vi "dfd_Expand Roots.vi"(1 "roots":T1[](array[typedef])) -> (0 "expanded roots":cdb[](array[numeric]))   [LabVIEW 2017, in "NI_DigFilterLicensed.lvlib"]
uses:
  <vilib>/addons/Digital Filter Design/NI_DigFilterLicensed.lvlib
  <vilib>/addons/Digital Filter Design/_Objects.llb/DFD Pole-Zero.ctl
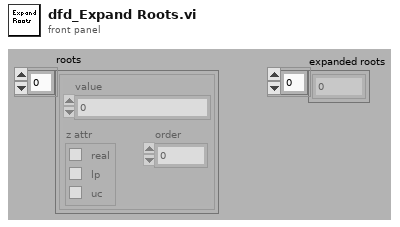
[diagram p1: front panel]
types:
  T1 = typedef "NI_DigFilterLicensed.lvlib/DFD Pole-Zero.ctl" = cluster{"value":cdb, "z attr":cluster{"real":bool, "lp":bool, "uc":bool}, "order":i32}
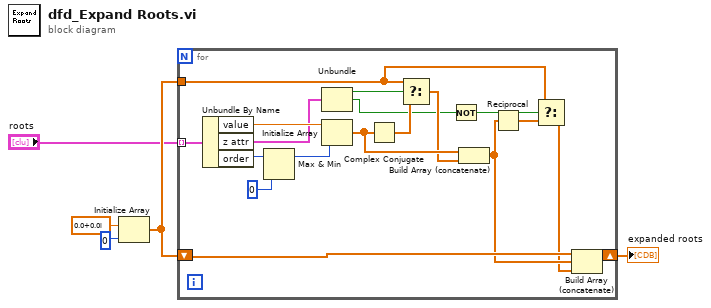
[diagram p0: block diagram]
diagram:
  n1 = Initialize Array(cdb 0.0+0.0i, 0) -> (w4:cdb[])
  n2 = for {
    shift-right: [w22] -> w5
    shift-left: w4 -> [w19]
    tunnel: "roots" -> [w23] mode=indexing
    tunnel: w4 -> [w8]
    n3 = Unbundle By Name(w23) -> ("value"=w18:cdb, "z attr"=w16:cluster{"real":bool, "lp":bool, "uc":bool}, "order"=w20:i32)
    n4 = Max & Min(x=w20, y=0) -> (max(x,y)=w17:i32)  [unwired: 1 out]
    n5 = Unbundle(w16) -> ("real"=w15:bool, "lp"=w11:bool)  [unwired: 1 out]
    n6 = Initialize Array(w18, w17) -> (w13:cdb[])
    n7 = Complex Conjugate(1:w13) -> (0:w14:cdb[])
    n8 = Select(t=w8, s=w15, f=w14) -> (s? t:f=w12:cdb[])
    n9 = Not(x=w11) -> (.not. x?=w10:bool)
    n10 = Build Array (concatenate)(w13, w12) -> (w7:cdb[])
    n11 = Reciprocal(x=w7) -> (1/x=w9:cdb[])
    n12 = Select(t=w8, s=w10, f=w9) -> (s? t:f=w6:cdb[])
    n13 = Build Array (concatenate)(w19, w7, w6) -> (w22:cdb[])
  }
  "expanded roots" <- w5
